vi "Measurement UI.vi"() -> ()   [LabVIEW 2021, in "Line Transient Response_PMIC_UI.lvlib"]
uses:
  Line Transient Response_PMIC_UI.lvlib
panel:
  in  "MeasGraphs":T1(tab)
  out "MeasTable":string[][](table)
  out "InputVoltageV/STimeGraph":waveform(dbl)(graph) caption="Load Transient"
  out "OutputVoltageV/STimeGraph":waveform(dbl)(graph) caption="Load Transient"
  in  "Source Voltage v/s Time":string="SOURCE VOLTAGE vs TIME"
  in  "Output Voltage v/s Time":string="LOAD VOLTAGE vs TIME"
  out "InputVoltageV/STimeGraphScope":waveform(dbl)(graph) caption="Load Transient"
  in  "ScopeSource Voltage v/s Time":string="SOURCE VOLTAGE vs TIME"
  out "OutputVoltageV/STimeScope":waveform(dbl)(graph) caption="Load Transient"
  in  "ScopeOutput Voltage v/s Time":string="LOAD VOLTAGE vs TIME"
  out "Overshoot load voltage":dbl
  out "Undershoot load voltage":dbl
  out "Scope amplitudes":dbl[](array[numeric])
  in  "Scope resource name":string
  in  "Load transient response":i32(ring)=1042 items=["Slow"=1041, "Normal"=1038, "Fast"=1039, "Custom"=1042]
  in  "Source resource name":string
  in  "Load resource name":string
  out "dt":dbl
  out "Load voltages":dbl[](array[numeric])
  out "Source voltages":dbl[](array[numeric])
  in  "Source transient response":i32(ring)=1042 items=["Slow"=1041, "Normal"=1038, "Fast"=1039, "Custom"=1042]
  in  "MeasConfigurations":enum32{"Source & Load Config", "Scope Config"}(tab)
  in  "Source update rate":dbl=1000.0 caption="UPDATE RATE" format="%#_6pS/s"
  in  "Load Sense":i32(ring)=1009 caption="LOAD SENSE" items=["Local"=1008, "Remote"=1009]
  in  "Source Sense":i32(ring)=1008 caption="SOURCE SENSE" items=["Local"=1008, "Remote"=1009]
  in  "Source voltage delay t2":dbl=0.005 caption="DELAY T2" format="%#_6ps"
  in  "Source voltage delay t1":dbl=0.005 caption="DELAY T1" format="%#_6ps"
  in  "Source voltatge pulse duration":dbl=0.005 caption="PULSE DURATION" format="%#_6ps"
  in  "Source voltage rising slew rate":dbl=1000.0 caption="VOLTAGE RISING SLEW RATE" format="%#_6pV/s"
  in  "Source voltage falling slew rate":dbl=1000.0 caption="VOLTAGE FALLING SLEW RATE" format="%#_6pV/s"
  in  "Source maximum power":dbl=300.0 caption="MAXIMUM POWER" format="%#_6pW"
  in  "Source current limit":dbl=0.25 caption="CURRENT LIMIT" format="%#_6pA"
  in  "Load configuration":string="Load configuration"
  in  "Source configuration":string="Source configuration"
  in  "Source voltage set point 2":dbl=20.0 caption="VOLTAGE SET POINT 2" format="%#_6pV"
  in  "Source voltage set point 1":dbl=7.0 caption="VOLTAGE SET POINT 1" format="%#_6pV"
  in  "PPSResourceName":refnum<k15> caption="RESOURCE NAME"
  in  "Source voltage pole-zero ratio":dbl=2.0 caption="POLE-ZERO RATIO"
  in  "Source voltage gain bandwidth":dbl=2000.0 caption="GAIN BANDWIDTH" format="%#_6pHz"
  in  "Source voltage compensation frequency":dbl=3530.0 caption="COMP. FREQUENCY" format="%#_6pHz"
  in  "Source fast":bool
  in  "Source normal":bool
  in  "Source slow":bool
  in  "Source SourceAdapt":string="Voltage SourceAdapt Parameters"
  in  "Load voltage limit range":dbl=4.0 caption="VOLTAGE LIMIT RANGE" format="%#_6pV"
  in  "Load current level range":dbl=4.0 caption="CURRENT LEVEL RANGE" format="%#_6pA"
  in  "Load current pole-zero ratio":dbl=0.3 caption="POLE-ZERO RATIO"
  in  "Load current gain bandwidth":dbl=14000.0 caption="GAIN BANDWIDTH" format="%#_6pHz"
  in  "Load current compensation frequency":dbl=180000.0 caption="COMP. FREQUENCY" format="%#_6pHz"
  in  "Source sample rate":dbl=1800000.0 caption="SAMPLE RATE" format="%#_6pS/s"
  in  "Load current level":dbl=0.03 caption="CURRENT LEVEL" format="%#_6pA"
  in  "ELOADResourceName":refnum<k15> caption="RESOURCE NAME"
  in  "Load fast":bool
  in  "Load normal":bool
  in  "Load slow":bool
  in  "Load SourceAdapt":string="Current SourceAdapt Parameters"
  in  "DUT setup time":dbl=1.0 caption="DUT SETUP TIME" format="%#_6ps"
  in  "Measurement settings":string="Measurement settings"
  in  "Nominal output voltage":dbl=3.3 caption="NOMINAL O/P VOLTAGE" format="%#_6pV"
  in  "Scope vertical range":dbl=10.0 caption="VERTICAL RANGE"
  out "Source status":string="Scope is enabled"
  in  "Scope enable/disable":bool=TRUE caption="Scope Enable/Disable"
  in  "SCOPEResourceName":refnum<k15> caption="RESOURCE NAME"
  in  "Scope probe attenuation":dbl=1.0 caption="PROBE ATTENUATION"
  in  "Scope sample rate":dbl=1800000.0 caption="SAMPLE RATE" format="%#_6pHz"
  in  "Scope output channel name":string="0" caption="OUTPUT CHANNEL NAME"
  in  "Scope vertical coupling":enum32{"AC", "DC"}(ring)=enum."DC" caption="VERTICAL COUPLING"
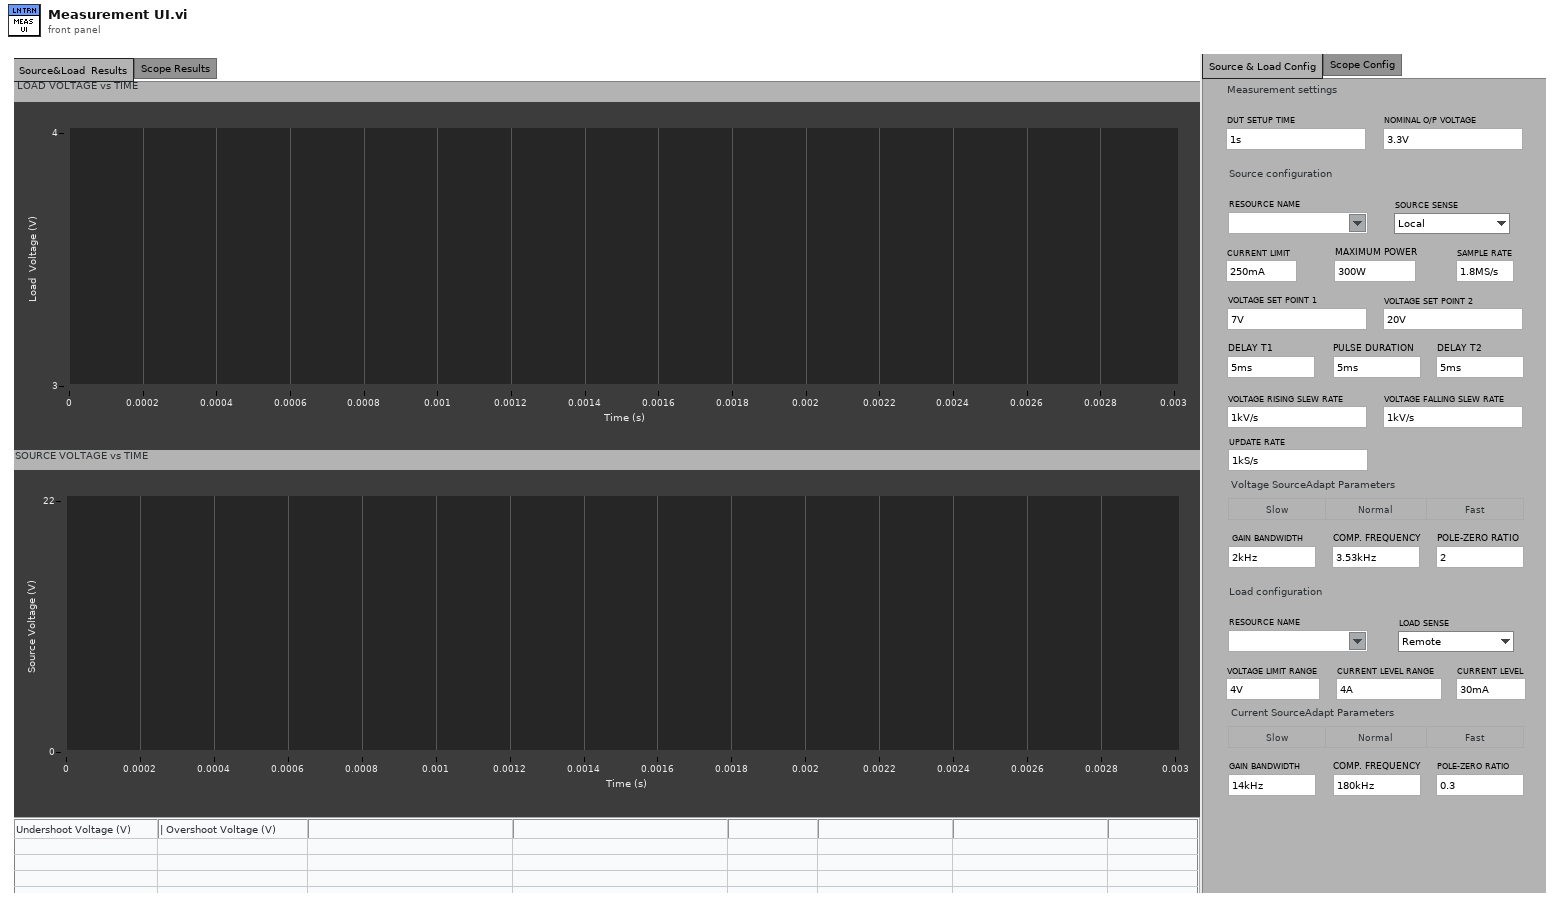
[diagram p1: front panel]
types:
  T1 = enum32{"Source&Load  Results", "Scope Results", "Hidden Controls"}
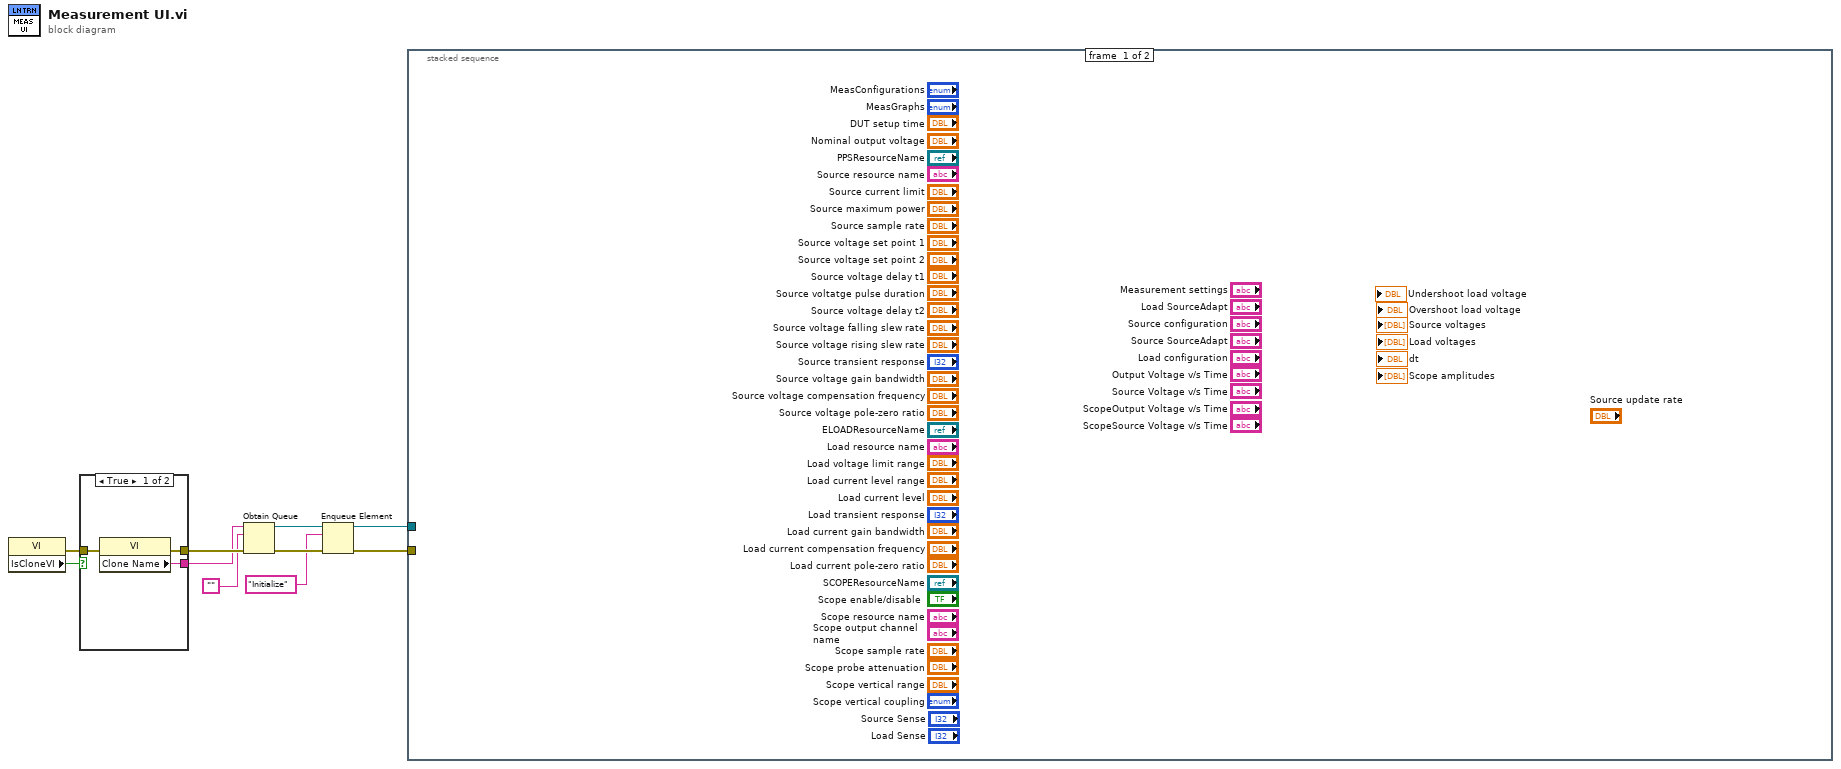
[diagram p0: block diagram]
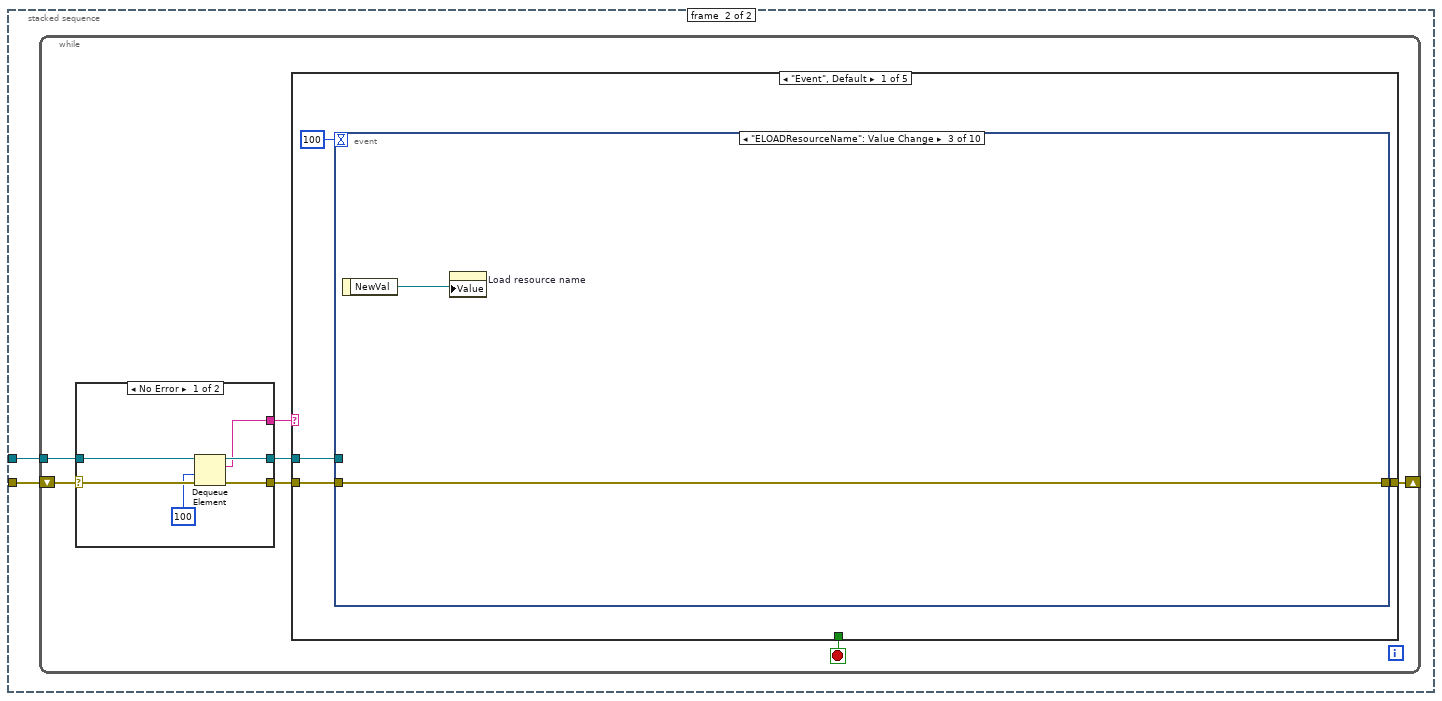
[diagram p2: hidden frame]
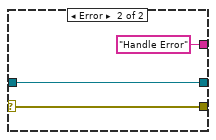
[diagram p3: hidden frame]
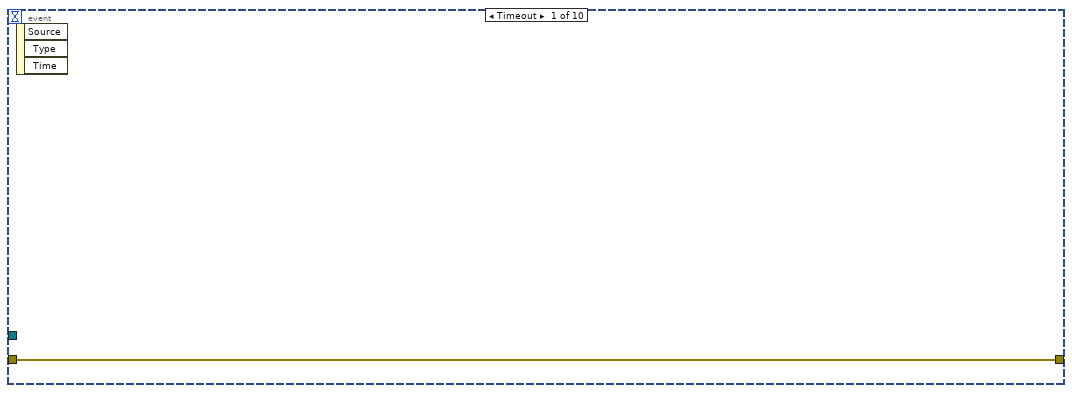
[diagram p4: hidden frame]
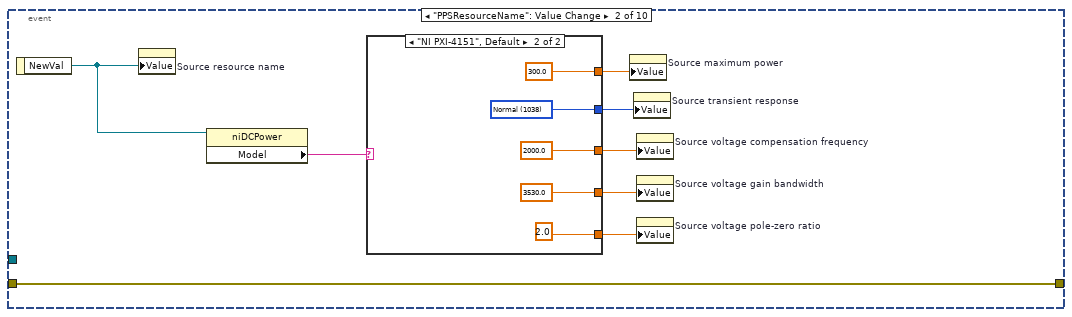
[diagram p5: hidden frame]
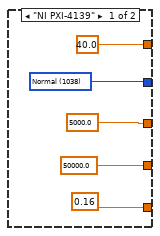
[diagram p6: hidden frame]
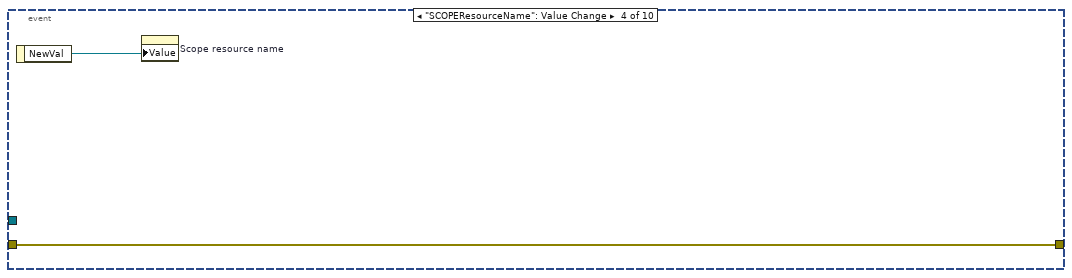
[diagram p7: hidden frame]
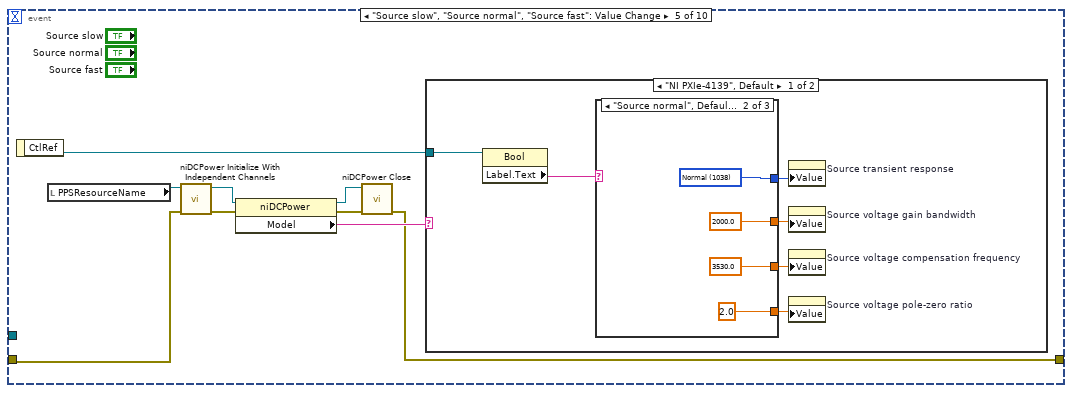
[diagram p8: hidden frame]
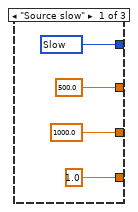
[diagram p9: hidden frame]
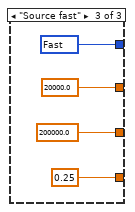
[diagram p10: hidden frame]
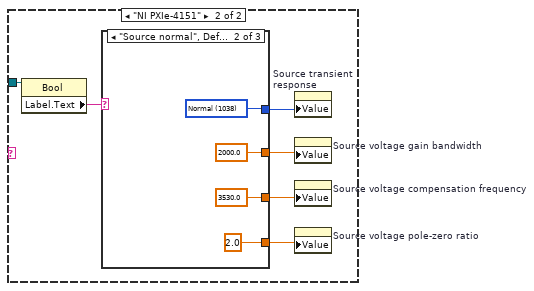
[diagram p11: hidden frame]
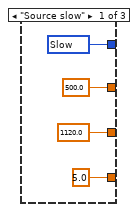
[diagram p12: hidden frame]
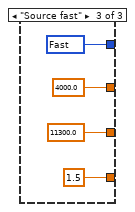
[diagram p13: hidden frame]
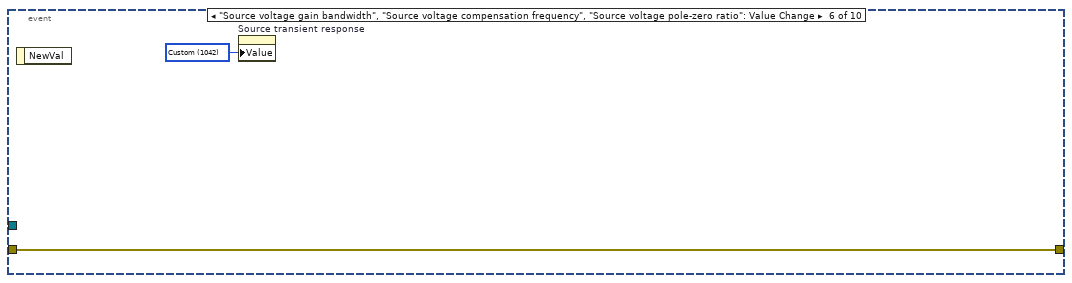
[diagram p14: hidden frame]
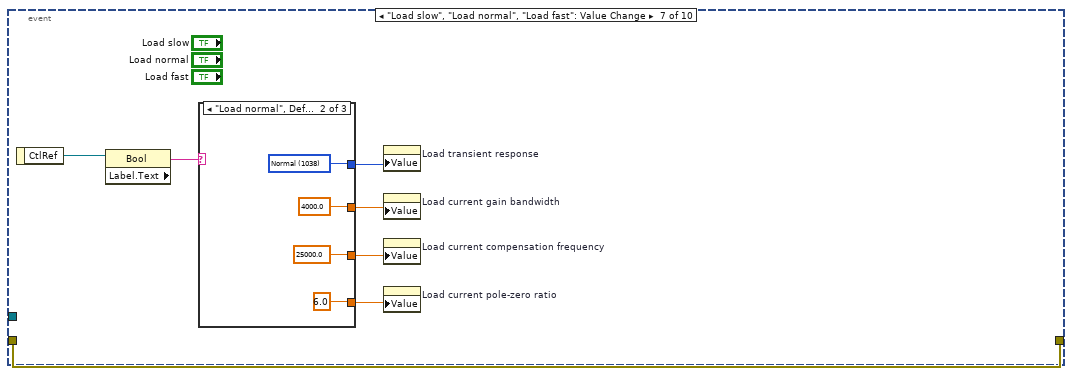
[diagram p15: hidden frame]
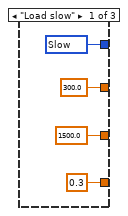
[diagram p16: hidden frame]
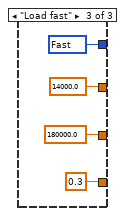
[diagram p17: hidden frame]
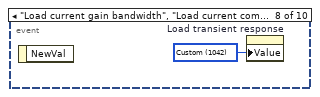
[diagram p18: hidden frame]
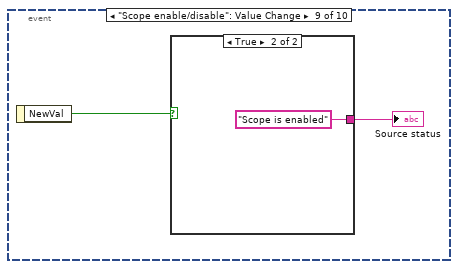
[diagram p19: hidden frame]
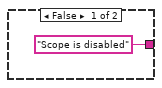
[diagram p20: hidden frame]
diagram:
  n1 = property class="VI"() -> (error out=w1:errorcluster, "IsCloneVI"=w2:bool)  [unwired: 2 in, 1 out]
  n2 = case shown="True" w2 {
    tunnel: [w13 w16] -> w10
    tunnel: [w12 w15] -> w9
    tunnel: w1 -> [w11 w14]
    frame True {
      n3 = property class="VI"(error in=w11) -> (error out=w13:errorcluster, "Clone Name"=w12:string)  [unwired: 1 in, 1 out]
    }
    frame False {
      n4 = property class="VI"(error in=w14) -> (error out=w16:errorcluster, "Name"=w15:string)  [unwired: 1 in, 1 out]
    }
  }
  n5 = Obtain Queue(name (unnamed)=w9, element data type="", error in (no error)=w10) -> (queue out=w6:refnum<queue>, error out=w8:errorcluster)  [unwired: 2 in, 1 out]
  n6 = Enqueue Element(queue=w6, element="Initialize", error in (no error)=w8) -> (queue out=w5:refnum<queue>, error out=w7:errorcluster)  [unwired: 1 in, 1 out]
  n7 = stacked-sequence {
    tunnel: w7 -> [_ w18]
    tunnel: w5 -> [_ w17]
    frame #0 {
    }
    frame #1 {
      n8 = while {
        shift-right: [w20] -> _
        shift-left: w18 -> [w25]
        tunnel: w17 -> [w23]
        stop <- w19 stop-if-true
        n9 = case shown="No Error" w25 {
          selector: w25 -> [w31 w34]
          tunnel: [w30 w34] -> w24
          tunnel: w23 -> [w29 w33]
          tunnel: [w28 w33] -> w22
          tunnel: [w27 "Handle Error"] -> w21
          frame No Error {
            n10 = Dequeue Element(queue=w29, timeout in ms (-1)=100, error in (no error)=w31) -> (queue out=w28:refnum<queue>, element=w27:string, error out=w30:errorcluster)  [unwired: 1 out]
          }
          frame Error {
          }
        }
        n11 = case shown="\"Event\", Default" w21 {
          tunnel: w24 -> [w37 w139 w159 w168 w169]
          tunnel: w22 -> [w35 _ _ w166 _]
          tunnel: [w38 w139 w159 w163 w169] -> w20
          tunnel: [_ FALSE _ TRUE _] -> w19
          frame "Event", Default {
            n12 = event shown="[2] \"ELOADResourceName\": Value Change" {
              selector: _ -> [_ _ _ _ _ _ _ _ _ _]
              dyn-events: _ -> [_ _ _ _ _ _ _ _ _ _]
              timeout: 100 -> [_ _ _ _ _ _ _ _ _ _]
              tunnel: [w39 w45 w58 w60 w62 w107 w109 _ _ w135] -> w38
              tunnel: w37 -> [w39 w45 w58 w60 w63 w107 w109 _ _ w136]
              tunnel: w35 -> [_ _ _ _ _ _ _ _ _ w134]
              event Timeout {
                n13 = event-data() -> ()  [unwired: 1 in, 3 out]
              }
              event "PPSResourceName": Value Change {
                n14 = event-data() -> ("NewVal"=w47:refnum<k15>)  [unwired: 1 in]
                n15 = property on="Source resource name" class="Str"("Value"=w47) -> ()  [unwired: 2 in, 2 out]
                n16 = property class="niDCPower"(reference=w47) -> ("Model"=w46:string)  [unwired: 1 in, 2 out]
                n17 = case shown="\"NI PXI-4151\", Default" w46 {
                  tunnel: [40.0 ("Source maximum power") 300.0 ("Source maximum power")] -> w44
                  tunnel: [w51 w56] -> w43
                  tunnel: [5000.0 ("Source maximum power") 2000.0 ("Source maximum power")] -> w42
                  tunnel: [50000.0 ("Source maximum power") 3530.0 ("Source maximum power")] -> w41
                  tunnel: [0.16 ("Source maximum power") 2.0 ("Source maximum power")] -> w40
                  frame "NI PXI-4139" {
                    w51 = 1038 items=["Slow"=1041, "Normal"=1038, "Fast"=1039, "Custom"=1042] ("Source transient response")
                  }
                  frame "NI PXI-4151", Default {
                    w56 = 1038 items=["Slow"=1041, "Normal"=1038, "Fast"=1039, "Custom"=1042] ("Source transient response")
                  }
                }
                n18 = property on="Source maximum power" class="DigNum (strict)"("Value"=w44) -> ()  [unwired: 2 in, 2 out]
                n19 = property on="Source transient response" class="Ring (strict)"("Value"=w43) -> ()  [unwired: 2 in, 2 out]
                n20 = property on="Source voltage compensation frequency" class="DigNum (strict)"("Value"=w42) -> ()  [unwired: 2 in, 2 out]
                n21 = property on="Source voltage gain bandwidth" class="DigNum (strict)"("Value"=w41) -> ()  [unwired: 2 in, 2 out]
                n22 = property on="Source voltage pole-zero ratio" class="DigNum (strict)"("Value"=w40) -> ()  [unwired: 2 in, 2 out]
              }
              event "ELOADResourceName": Value Change {
                n23 = event-data() -> ("NewVal"=w59:refnum<k15>)  [unwired: 1 in]
                n24 = property on="Load resource name" class="Str"("Value"=w59) -> ()  [unwired: 2 in, 2 out]
              }
              event "SCOPEResourceName": Value Change {
                n25 = event-data() -> ("NewVal"=w61:refnum<k15>)  [unwired: 1 in]
                n26 = property on="Scope resource name" class="Str"("Value"=w61) -> ()  [unwired: 2 in, 2 out]
              }
              event "Source slow", "Source normal", "Source fast": Value Change {
                n27 = event-data() -> ("CtlRef"=w70:refnum<vi>)  [unwired: 1 in]
                n28 = local read "PPSResourceName"() -> (w68:refnum<k15>)
                n29 = call <instrlib>:"niDCPower Initialize With Independent Channels.vi"("error in (no error)"=w63, "resource name"=w68) -> ("error out"=w65:errorcluster, "instrument handle out"=w67:refnum<k15>)  [unwired: 8 in]
                n30 = property class="niDCPower"(reference=w67, error in=w65) -> (reference out=w66:refnum<k15>, error out=w64:errorcluster, "Model"=w69:string)
                n31 = call <instrlib>:"niDCPower Close.vi"("error in (no error)"=w64, "instrument handle"=w66) -> ("error out"=w62:errorcluster)  [unwired: 9 in]
                n32 = case shown="\"NI PXIe-4139\", Default" w69 {
                  tunnel: w70 -> [w71 w89]
                  frame "NI PXIe-4139", Default {
                    n33 = property class="Bool"(reference=w71) -> ("Label.Text"=w76:string)  [unwired: 1 in, 2 out]
                    n34 = case shown="\"Source normal\", Default" w76 {
                      tunnel: [w80 w84 w88] -> w75
                      tunnel: [500.0 ("Source voltage gain bandwidth") 2000.0 ("Source voltage gain bandwidth") 20000.0 ("Source voltage gain bandwidth")] -> w74
                      tunnel: [1000.0 ("Source voltage compensation frequency") 3530.0 ("Source voltage compensation frequency") 200000.0 ("Source voltage compensation frequency")] -> w73
                      tunnel: [1.0 ("Source voltage pole-zero ratio") 2.0 ("Source voltage pole-zero ratio") 0.25 ("Source voltage pole-zero ratio")] -> w72
                      frame "Source slow" {
                        w80 = 1041 items=["Slow"=1041, "Normal"=1038, "Fast"=1039, "Custom"=1042] ("Source transient response")
                      }
                      frame "Source normal", Default {
                        w84 = 1038 items=["Slow"=1041, "Normal"=1038, "Fast"=1039, "Custom"=1042] ("Source transient response")
                      }
                      frame "Source fast" {
                        w88 = 1039 items=["Slow"=1041, "Normal"=1038, "Fast"=1039, "Custom"=1042] ("Source transient response")
                      }
                    }
                    n35 = property on="Source transient response" class="Ring (strict)"("Value"=w75) -> ()  [unwired: 2 in, 2 out]
                    n36 = property on="Source voltage gain bandwidth" class="DigNum (strict)"("Value"=w74) -> ()  [unwired: 2 in, 2 out]
                    n37 = property on="Source voltage compensation frequency" class="DigNum (strict)"("Value"=w73) -> ()  [unwired: 2 in, 2 out]
                    n38 = property on="Source voltage pole-zero ratio" class="DigNum (strict)"("Value"=w72) -> ()  [unwired: 2 in, 2 out]
                  }
                  frame "NI PXIe-4151" {
                    n39 = property class="Bool"(reference=w89) -> ("Label.Text"=w94:string)  [unwired: 1 in, 2 out]
                    n40 = case shown="\"Source normal\", Default" w94 {
                      tunnel: [w98 w102 w106] -> w93
                      tunnel: [500.0 ("Source voltage gain bandwidth") 2000.0 ("Source voltage gain bandwidth") 4000.0 ("Source voltage gain bandwidth")] -> w92
                      tunnel: [1120.0 ("Source voltage compensation frequency") 3530.0 ("Source voltage compensation frequency") 11300.0 ("Source voltage compensation frequency")] -> w91
                      tunnel: [5.0 ("Source voltage pole-zero ratio") 2.0 ("Source voltage pole-zero ratio") 1.5 ("Source voltage pole-zero ratio")] -> w90
                      frame "Source slow" {
                        w98 = 1041 items=["Slow"=1041, "Normal"=1038, "Fast"=1039, "Custom"=1042] ("Source transient response")
                      }
                      frame "Source normal", Default {
                        w102 = 1038 items=["Slow"=1041, "Normal"=1038, "Fast"=1039, "Custom"=1042] ("Source transient response")
                      }
                      frame "Source fast" {
                        w106 = 1039 items=["Slow"=1041, "Normal"=1038, "Fast"=1039, "Custom"=1042] ("Source transient response")
                      }
                    }
                    n41 = property on="Source transient response" class="Ring (strict)"("Value"=w93) -> ()  [unwired: 2 in, 2 out]
                    n42 = property on="Source voltage gain bandwidth" class="DigNum (strict)"("Value"=w92) -> ()  [unwired: 2 in, 2 out]
                    n43 = property on="Source voltage compensation frequency" class="DigNum (strict)"("Value"=w91) -> ()  [unwired: 2 in, 2 out]
                    n44 = property on="Source voltage pole-zero ratio" class="DigNum (strict)"("Value"=w90) -> ()  [unwired: 2 in, 2 out]
                  }
                }
              }
              event "Source voltage gain bandwidth", "Source voltage compensation frequency", "Source voltage pole-zero ratio": Value Change {
                w108 = 1042 items=["Slow"=1041, "Normal"=1038, "Fast"=1039, "Custom"=1042] ("Source transient response")
                n45 = event-data() -> ()  [unwired: 1 in, 1 out]
                n46 = property on="Source transient response" class="Ring (strict)"("Value"=w108) -> ()  [unwired: 2 in, 2 out]
              }
              event "Load slow", "Load normal", "Load fast": Value Change {
                n47 = event-data() -> ("CtlRef"=w110:refnum<vi>)  [unwired: 1 in]
                n48 = property class="Bool"(reference=w110) -> ("Label.Text"=w115:string)  [unwired: 1 in, 2 out]
                n49 = case shown="\"Load normal\", Default" w115 {
                  tunnel: [w119 w123 w127] -> w114
                  tunnel: [300.0 ("Load current gain bandwidth") 4000.0 ("Load current gain bandwidth") 14000.0 ("Load current gain bandwidth")] -> w113
                  tunnel: [1500.0 ("Load current compensation frequency") 25000.0 ("Load current compensation frequency") 180000.0 ("Load current compensation frequency")] -> w112
                  tunnel: [0.3 ("Load current pole-zero ratio") 6.0 ("Load current pole-zero ratio") 0.3 ("Load current pole-zero ratio")] -> w111
                  frame "Load slow" {
                    w119 = 1041 items=["Slow"=1041, "Normal"=1038, "Fast"=1039, "Custom"=1042] ("Source transient response")
                  }
                  frame "Load normal", Default {
                    w123 = 1038 items=["Slow"=1041, "Normal"=1038, "Fast"=1039, "Custom"=1042] ("Source transient response")
                  }
                  frame "Load fast" {
                    w127 = 1039 items=["Slow"=1041, "Normal"=1038, "Fast"=1039, "Custom"=1042] ("Source transient response")
                  }
                }
                n50 = property on="Load transient response" class="Ring (strict)"("Value"=w114) -> ()  [unwired: 2 in, 2 out]
                n51 = property on="Load current gain bandwidth" class="DigNum (strict)"("Value"=w113) -> ()  [unwired: 2 in, 2 out]
                n52 = property on="Load current compensation frequency" class="DigNum (strict)"("Value"=w112) -> ()  [unwired: 2 in, 2 out]
                n53 = property on="Load current pole-zero ratio" class="DigNum (strict)"("Value"=w111) -> ()  [unwired: 2 in, 2 out]
              }
              event "Load current gain bandwidth", "Load current compensation frequency", "Load current pole-zero ratio": Value Change {
                w128 = 1042 items=["Slow"=1041, "Normal"=1038, "Fast"=1039, "Custom"=1042] ("Load transient response")
                n54 = event-data() -> ()  [unwired: 1 in, 1 out]
                n55 = property on="Load transient response" class="Ring (strict)"("Value"=w128) -> ()  [unwired: 2 in, 2 out]
              }
              event "Scope enable/disable": Value Change {
                n56 = event-data() -> ("NewVal"=w130:bool)  [unwired: 1 in]
                n57 = case shown="True" w130 {
                  tunnel: ["Scope is disabled" ("Load status") "Scope is enabled" ("Load status")] -> w129
                  frame False {
                  }
                  frame True {
                  }
                }
                "Source status" <- w129
              }
              event Panel Close? {
                n58 = event-data() -> ()  [unwired: 1 in, 4 out]
                n59 = Enqueue Element(queue=w134, element="Exit", error in (no error)=w136) -> (error out=w135:errorcluster)  [unwired: 1 in, 2 out]
                n60 = event-data("Discard?"=TRUE) -> ()  [unwired: 1 in, 1 out]
              }
            }
          }
          frame "Initialize" {
          }
          frame "Post UI Update" {
            # "This case will be triggered, after framework updates the User interface with result values."
            n61 = local read "Scope enable/disable"() -> (w152:bool)
            n62 = local read "Scope amplitudes"() -> (w154:dbl[])
            n63 = local read "Source voltages"() -> (w151:dbl[])
            n64 = local read "Load voltages"() -> (w158:dbl[])
            n65 = local read "dt"() -> (w148:dbl)
            n66 = case shown="True" w152 {
              tunnel: w151 -> [_ w161]
              tunnel: [dbl[] [] ("Source voltages") w161] -> w150
              frame False {
              }
              frame True {
              }
            }
            n67 = Bundle By Name("dt"=w148, "Y"=w154) -> (→"OutputVoltageV/STimeScope":waveform(dbl))  [unwired: 1 in]
            n68 = Bundle By Name("Y"=w158, "dt"=w148) -> (→"OutputVoltageV/STimeGraph":waveform(dbl))  [unwired: 1 in]
            n69 = Bundle By Name("dt"=w148, "Y"=w151) -> (→"InputVoltageV/STimeGraph":waveform(dbl))  [unwired: 1 in]
            n70 = local read "Undershoot load voltage"() -> (w144:dbl)
            n71 = local read "Overshoot load voltage"() -> (w143:dbl)
            n72 = Bundle By Name("dt"=w148, "Y"=w150) -> (→"InputVoltageV/STimeGraphScope":waveform(dbl))  [unwired: 1 in]
            n73 = Format Into String(format string="%.3f" ("initial string"), initial string="|   ", w143) -> (resulting string=w142:string)  [unwired: 1 in, 1 out]
            n74 = Format Into String(format string="%.3f" ("initial string"), w144) -> (resulting string=w149:string)  [unwired: 2 in, 1 out]
            n75 = Build Array(w149, w142) -> (w141:string[])
            n76 = Build Array(w141) -> (→"MeasTable":string[][])
          }
          frame "Exit" {
            # "This case is triggered to close the User Interface from framework"
            n77 = Flush Queue(queue=w166, error in (no error)=w168) -> (queue out=w165:refnum<queue>, error out=w164:errorcluster)  [unwired: 1 out]
            n78 = Release Queue(queue=w165, force destroy? (F)=TRUE, error in (no error)=w164) -> (error out=w163:errorcluster)  [unwired: 2 out]
          }
          frame "Handle Error" {
          }
        }
      }
    }
  }
